vi "Out_S1F16.vi"(8 "error in (no error)":errorcluster, 10 "Ack":bool, 11 "S1 Message Class in":refnum<class "S1 Message Class.lvclass">) -> (0 "error out":errorcluster, 3 "S1 Message Class out":refnum<class "S1 Message Class.lvclass">)   [LabVIEW 2020, in "SECS Communication.lvlib" / "S1 Message Class.lvclass"]
uses:
  S1 Message Class.lvclass
  D:/Dropbox/SECS/LabVIEW Code/Com/SECS Communication/SECS-II Class/SECS-II Class.lvclass
  SECS-II Class/Data Message_Binary.vi
  S1 Message Class.lvclass/S1 Message Class.ctl
  SECS-II Class/SECS-II Class.lvclass
  D:/Dropbox/SECS/LabVIEW Code/Com/SECS Communication/S1 Message Class/S1 Message Class.lvclass
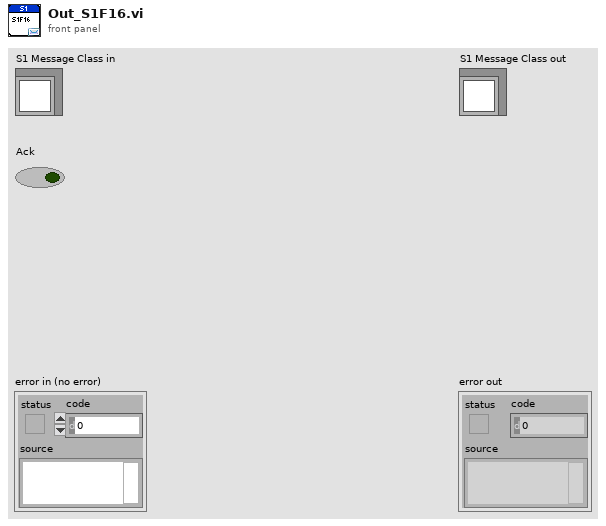
[diagram p1: front panel]
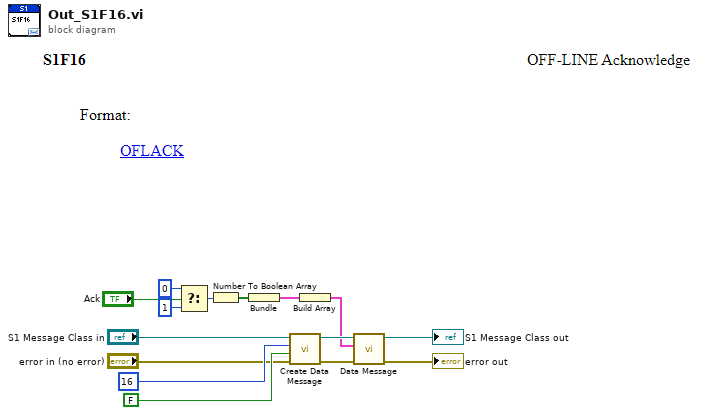
[diagram p0: block diagram]
diagram:
  n1 = Select(t=u8 0, s="Ack", f=u8 1) -> (s? t:f=w1:u8)
  n2 = Number To Boolean Array(number=w1) -> (Boolean array=w7:bool[])
  n3 = Bundle("Boolean array"=w7) -> (w6:cluster{"Boolean array":bool[]})  [unwired: 1 in]
  n4 = call "Create Data Message.vi"("error in (no error)"="error in (no error)", "W-Bit"=FALSE, "Function"=u8 16, "SECS-II Class in"="S1 Message Class in") -> ("error out"=w10:errorcluster, "SECS-II Class out"=w11:refnum<class "S1 Message Class.lvclass">)  [unwired: 6 in]
  n5 = Build Array(w6) -> (w5:cluster{"Boolean array":bool[]}[])
  n6 = call-poly "Data Message.vi"("error in"=w10, "Data Cluster"=w5, "SECS-II Class in"=w11) -> ("error out"=→"error out":errorcluster, "SECS-II Class out"=→"S1 Message Class out":refnum<class "S1 Message Class.lvclass">)  [unwired: 7 in]
